vi "ATF Storage-ACC Start.vi"(8 "error in":errorcluster, 9 "ACC config":T1(array[cluster]), 11 "Refnum in":refnum<k21>) -> (0 "error out":errorcluster, 3 "Refnum out":refnum<k21>)   [LabVIEW 2022 SP3]
doc: "This VI is for TC Start task"
uses:
  <vilib>/DAQmx/configure/timing.llb/DAQmx Timing (Sample Clock).vi
  <vilib>/DAQmx/configure/trigger.llb/DAQmx Start Trigger (Digital Edge).vi
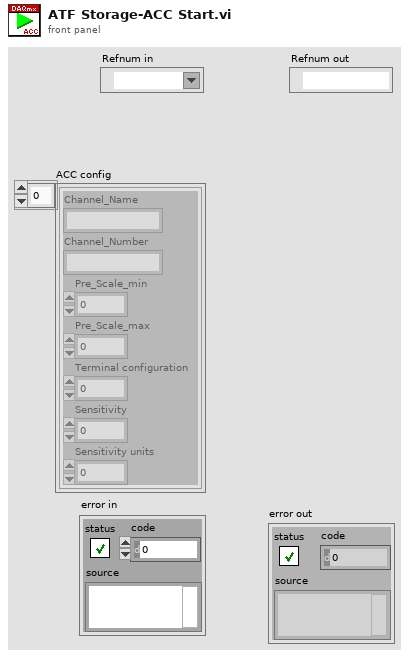
[diagram p1: front panel]
types:
  T1 = cluster{"Channel_Name":string, "Channel_Number":string, "Pre_Scale_min":dbl, "Pre_Scale_max":dbl, "Terminal configuration":i32, "Sensitivity":dbl, "Sensitivity units":i32}[]
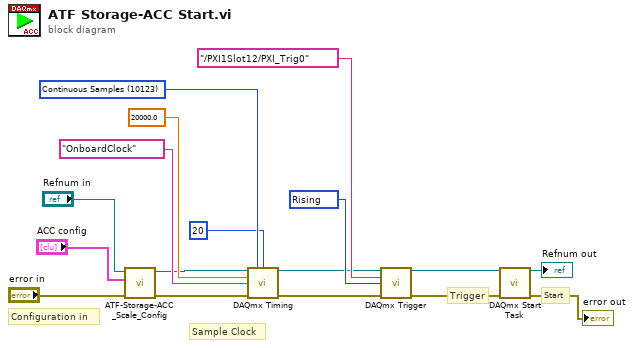
[diagram p0: block diagram]
diagram:
  w6 = 10280 items=["Rising"=10280, "Falling"=10171] ("edge")
  w14 = 10123 items=["Finite Samples"=10178, "Continuous Samples"=10123, "Hardware Timed Single Point"=12522] ("sample mode")
  # "Start"
  # "Trigger"
  # "Sample Clock"
  # "Configuration in"
  n1 = call "ATF-Storage-ACC_Scale_Config.vi"("error in (no error)"="error in", "ACC config"="ACC config", "Refnum in"="Refnum in") -> ("error out"=w10:errorcluster, "Refnum out"=w7:refnum<k21>)  [unwired: 7 in]
  n2 = call-poly <vilib>:"DAQmx Timing.vi"("task/channels in"=w7, "sample mode"=w14, "samples per channel"=20, "rate"=20000.0, "source"=tag "OnboardClock", "error in"=w10) -> ("task out"=w4:refnum<k21>, "error out"=w2:errorcluster)  [unwired: 8 in]
  n3 = call-poly <vilib>:"DAQmx Trigger.vi"("task/channels in"=w4, "source"=tag "/PXI1Slot12/PXI_Trig0", "edge"=w6, "error in"=w2) -> ("task out"=w3:refnum<k21>, "error out"=w1:errorcluster)  [unwired: 10 in]
  n4 = call <vilib>:"DAQmx Start Task.vi"("task/channels in"=w3, "error in"=w1) -> ("task out"=→"Refnum out":refnum<k21>, "error out"=→"error out":errorcluster)  [unwired: 12 in]
